vi "Import Permanent Variable From File.vi"(8 "error in (no error)":errorcluster, 9 "section postfix":string, 10 "Path":path, 11 "CSM-Static-Variable-Manager in":refnum<class "CSM-Static-Variable-Manager.lvclass">) -> (0 "error out":errorcluster, 3 "CSM-Static-Variable-Manager out":refnum<class "CSM-Static-Variable-Manager.lvclass">)   [LabVIEW 2017, in "INI-Static-Variable-Support.lvlib" / "CSM-Static-Variable-Manager.lvclass"]
uses:
  CSM-Static-Variable-Manager.lvclass
  CSM-Static-Variable-Manager.lvclass/CSM-Static-Variable-Manager.ctl
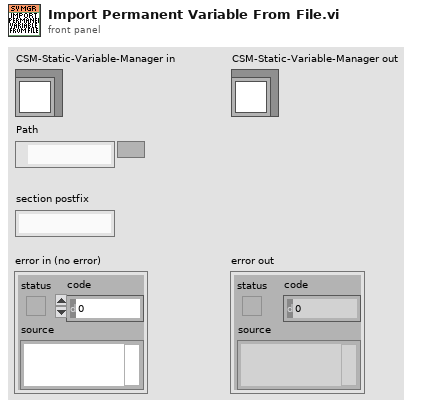
[diagram p1: front panel]
types:
  T1 = cluster{"Variable-FileMap":variant, "FileConfigMap":variant, "Memory":refnum<class "LabVIEW-Config.lvclass">}
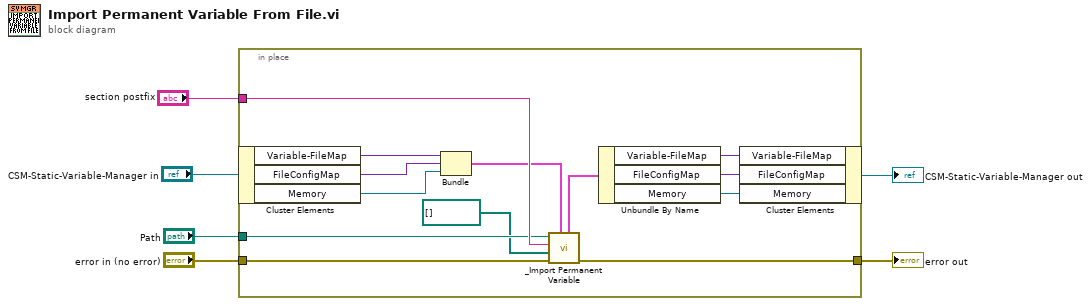
[diagram p0: block diagram]
diagram:
  n1 = in-place {
    in-place-border: "Path" -> [w16]
    in-place-border: "error in (no error)" -> [w17]
    in-place-border: [w18] -> w2
    in-place-border: "section postfix" -> [w19]
    n2 = in-place-cluster #1("CSM-Static-Variable-Manager in") -> ("Variable-FileMap"=w15:variant, "FileConfigMap"=w14:variant, "Memory"=w13:refnum<class "LabVIEW-Config.lvclass">)
    n3 = Bundle("Variable-FileMap"=w15, "FileConfigMap"=w14, "Memory"=w13) -> (w12:T1)  [unwired: 1 in]
    n4 = call "_Import Permanent Variable.vi"("in"=w12, "error in (no error)"=w17, "Array"=path[] [], "section postfix"=w19, "Path"=w16) -> ("error out"=w18:errorcluster, "out"=w11:T1)  [unwired: 5 in]
    n5 = Unbundle By Name(w11) -> ("Variable-FileMap"=w10:variant, "FileConfigMap"=w9:variant, "Memory"=w8:refnum<class "LabVIEW-Config.lvclass">)
    n6 = in-place-cluster #1("Variable-FileMap"=w10, "FileConfigMap"=w9, "Memory"=w8) -> (→"CSM-Static-Variable-Manager out":refnum<class "CSM-Static-Variable-Manager.lvclass">)
  }
  "error out" <- w2
